vi "Set Setting.vi"(0 "Setting name":string, 5 "Setting value":string, 11 "error in (no error)":errorcluster) -> (4 "Setting value out":string, 6 "Setting already included":bool, 15 "error out":errorcluster)   [LabVIEW 2023, in "RFCalAndFixtureCharact.Common.lvlib"]
uses:
  RFCalAndFixtureCharact.Common.lvlib
  Type Definitions/Dictionary Operation.ctl
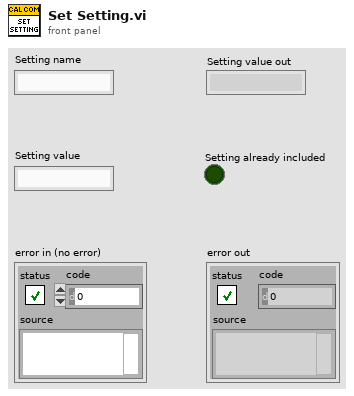
[diagram p1: front panel]
types:
  T1 = typedef "RFCalAndFixtureCharact.Common.lvlib/Dictionary Operation.ctl" = enum16{"Read", "Insert", "Remove", "Clear", "Get All", "Update"}
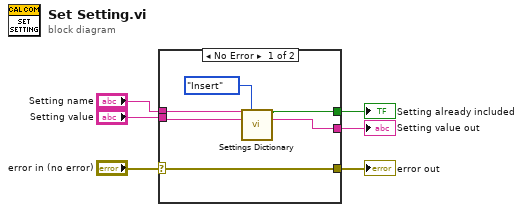
[diagram p0: block diagram]
diagram:
  n1 = case shown="No Error" "error in (no error)" {
    selector: "error in (no error)" -> [w12 w13]
    tunnel: "Setting name" -> [w10 _]
    tunnel: "Setting value" -> [w9 _]
    tunnel: [w7 _] -> w4
    tunnel: [w12 w13] -> w2
    tunnel: [w8 _] -> w1
    frame No Error {
      n2 = call "Settings Dictionary.vi"("Setting name"=w10, "Action"=Dictionary_Operation."Insert", "Setting value"=w9) -> ("Setting already included? / Setting not found?"=w8:bool, "Setting value out"=w7:string)  [unwired: 11 in]
    }
    frame Error {
    }
  }
  "error out" <- w2
  "Setting value out" <- w4
  "Setting already included" <- w1
